vi "Measurements 2 Target Arrays.vi"(10 "LBCB Command Data":T3[](array[typedef]), 11 "Target  Inputs":T1[](array[typedef])) -> (3 "Target  Outputs":T1[](array[typedef]))   [LabVIEW 2013]
uses:
  MixedMode/Mixed Mode Cartesian Data.ctl
  MixedMode/Messages/Target.ctl
  Data Access Objects/Metadata/LBCB Number.ctl
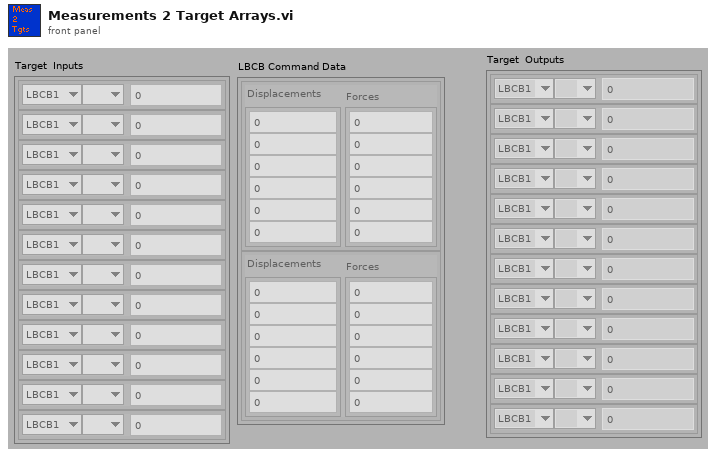
[diagram p1: front panel]
types:
  T1 = typedef "Target.ctl" = cluster{"LBCB Number":T2, "DOF Vectors":enum16{" ", "Dx", "Dy", "Dz", "Rx", "Ry", "Rz", "Fx", "Fy", "Fz", "Mx", "My", "Mz"}, "Amount":dbl}
  T2 = typedef "LBCB Number.ctl" = enum16{"LBCB1", "LBCB2"}
  T3 = typedef "Mixed Mode Cartesian Data.ctl" = cluster{"Displacements":dbl[], "Forces":dbl[]}
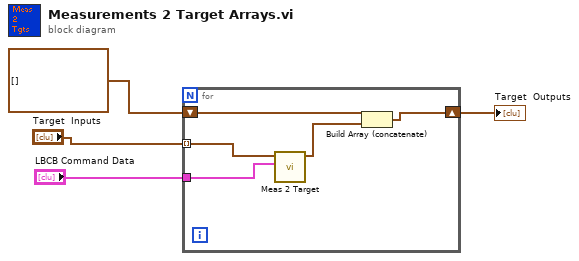
[diagram p0: block diagram]
diagram:
  n1 = for {
    tunnel: "Target  Inputs" -> [w9] mode=indexing
    shift-right: [w5] -> w1
    shift-left: T1[] [] -> [w6]
    tunnel: "LBCB Command Data" -> [w8]
    n2 = call "Meas 2 Target.vi"("LBCB  Data"=w8, "Target"=w9) -> ("Measured Value"=w7:T1)  [unwired: 2 in, 7 out]
    n3 = Build Array (concatenate)(w6, w7) -> (w5:T1[])
  }
  "Target  Outputs" <- w1
